vi "Assert String Not Contains String Ignoring Case.vi"(5 "Needle":string, 7 "Message (\"\")":string, 8 "error in (no error)":errorcluster, 10 "Haystack":string) -> (0 "error out":errorcluster)   [LabVIEW 2017, in "Assertion.lvlib"]
doc: "Asserts that <B>haystack</B> does not contain <B>needle</B>. Ignores differences in casing. Does nothing if an error occurred before this node runs. Returns an error if the assertion failed. Optionally adds a message to the error message if the assertion failed."
uses:
  Assertion.lvlib
  Constraint/LogicalNot/LogicalNot.lvclass
  Constraint/StringContains/StringContains.lvclass
  C:/Users/de200256/Code/logmanoriginal/lvunit/Constraint/Constraint/Constraint.lvclass
  Constraint/UnaryOperator/UnaryOperator.lvclass
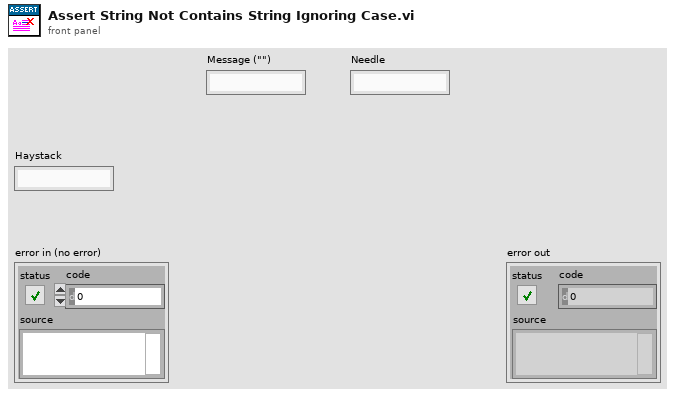
[diagram p1: front panel]
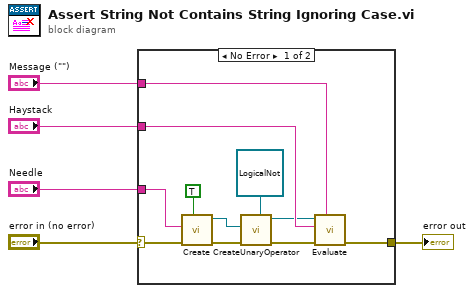
[diagram p0: block diagram]
diagram:
  n1 = case shown="No Error" "error in (no error)" {
    selector: "error in (no error)" -> [w12 w17]
    tunnel: "Haystack" -> [w15 _]
    tunnel: [w14 w17] -> w4
    tunnel: "Message (\"\")" -> [w13 _]
    tunnel: "Needle" -> [w11 _]
    frame No Error {
      n2 = call "Create.vi"("Ignore Case (F)"=TRUE, "error in (no error)"=w12, "Needle"=w11) -> ("error out"=w16:errorcluster, "StringContains"=w8:refnum<class "StringContains.lvclass">)  [unwired: 7 in]
      n3 = call-dynamic "CreateUnaryOperator.vi"("UnaryOperator In"=refnum<class "LogicalNot.lvclass"> refnum ("Constraint.lvlib:LogicalNot.lvclass"), "error in (no error)"=w16, "Constraint"=w8) -> ("error out"=w9:errorcluster, "UnaryOperator"=w7:refnum<class "UnaryOperator.lvclass">)  [unwired: 7 in]
      n4 = call-dynamic "Evaluate.vi"("Message (\"\")"=w13, "error in (no error)"=w9, "Actual"=w15, "Constraint in"=w7) -> ("error out"=w14:errorcluster)  [unwired: 6 in, 1 out]
    }
    frame Error {
    }
  }
  "error out" <- w4
